vi "As Bytes.vi"(11 "UUID in":refnum<class "UUID.lvclass">) -> (3 "Bytes":u8[](array[numeric]))   [LabVIEW 2015, in "UUID.lvclass"]
uses:
  UUID.lvclass
  UUID.lvclass/UUID.ctl
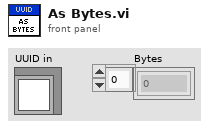
[diagram p1: front panel]
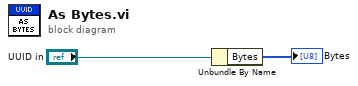
[diagram p0: block diagram]
diagram:
  n1 = Unbundle By Name("UUID in") -> ("Bytes"=→"Bytes":u8[])
